vi "HTSuperProWriteControl.vi"(0 "Digital Control":u8, 3 "NXT":T1={"error"={"status"=FALSE, "code"=0, "source"=""}, "address"="", "NXT #"=-1, "Show Error"=TRUE, "Connection"=4} {"Connection" items=["USB", "Bluetooth", "USB then Bluetooth", "Last Connection", "Preference"]}, 4 "Port":T2 items=["Port 1", "Port 2", "Port 3", "Port 4"]) -> (5 "NXT":T1={"error"={"status"=FALSE, "code"=0, "source"=""}, "address"="", "NXT #"=-1, "Show Error"=TRUE, "Connection"=4} {"Connection" items=["USB", "Bluetooth", "USB then Bluetooth", "Last Connection", "Preference"]})   [LabVIEW 2009]
doc: "HiTechnic SuperPro - Write Control\n\n<B>Inputs\nPort </B> is the port connected to the sensor. Port 1 is the default, but Port 2, Port 3, or Port 4 can also be selected.\n<B>NXT </B> connects to NXT terminal of previous VI to establish the flow of the program.\n<B>Digital Control</B> bits set to 1 in the Digital Control will configure corresponding output B0-B7 pins as output. By default all pins on the SuperPro are set for input.\n\n<B>Outputs\nNXT </B> wires to NXT terminal of next VI to establish the flow of the program."
uses:
  <vilib>/NXT/Block Support/NXT_InputPort.ctl
  <vilib>/NXT/Subs/LVHSConnector.ctl
  <vilib>/NXT/Block Support/HWPage.SensorType.ctl
  <vilib>/NXT/Block Support/HWPage.SensorMode.ctl
panel:
  # "HiTechnic SuperPro Prototype board VI\nWrite Control\n\nBits set to 1 in the Digital Control will configure corresponding output B0-B7 pins as output.   By default all pins on the SuperPro are set for input.\n\n(c) HiTechnic 2011"
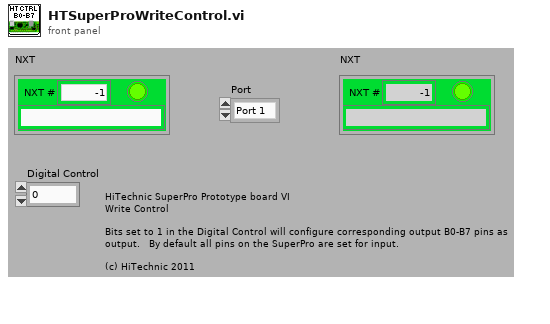
[diagram p1: front panel]
types:
  T1 = typedef "LVHSConnector.ctl" = cluster{"error":errorcluster, "address":string, "NXT #":i32, "Show Error":bool, "Connection":u16}
  T2 = typedef "NXT_InputPort.ctl" = u8
  T3 = typedef "HWPage.SensorType.ctl" = u8
  T4 = typedef "HWPage.SensorMode.ctl" = u8
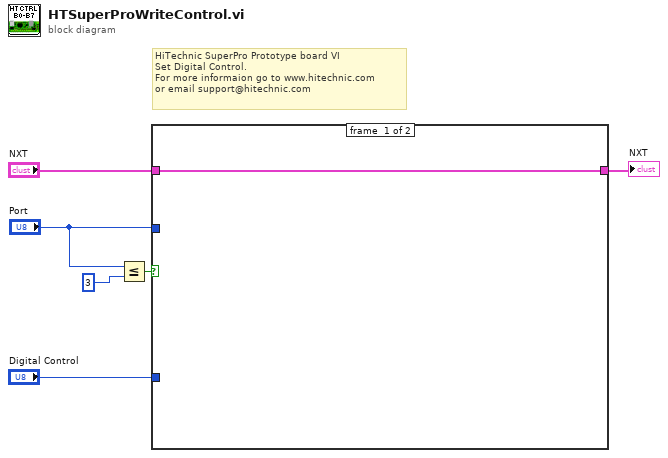
[diagram p0: block diagram]
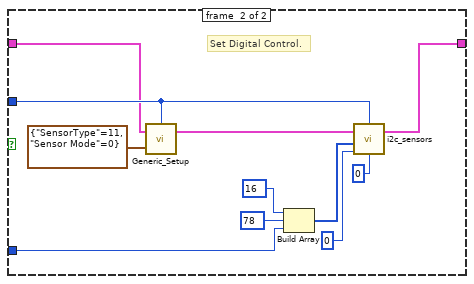
[diagram p2: hidden frame]
diagram:
  # "HiTechnic SuperPro Prototype board VI\nSet Digital Control.\nFor more informaion go to www.hitechnic.com\nor email support@hitechnic.com"
  n1 = Less Or Equal?(x="Port", y=u8 3) -> (x <= y?=w2:bool)
  n2 = case shown="True" w2 {
    tunnel: "Port" -> [_ w17]
    tunnel: "NXT" -> [w7 w16]
    tunnel: [w7 w14] -> w4
    tunnel: "Digital Control" -> [_ w9]
    frame #0 {
    }
    frame #1 {
      # "Set Digital Control."
      n3 = call <vilib>:"Generic_Setup.vi"("Sensor Setup"=cluster{"SensorType":T3, "Sensor Mode":T4} {"SensorType"=11, "Sensor Mode"=0}, "NXT"=w16, "Port"=w17) -> ("NXT"=w15:T1)  [unwired: 1 out]
      n4 = Build Array(u8 16, u8 78, w9) -> (w12:u8[])
      n5 = call <vilib>:"i2c_sensors.vi"("Return Length"=u8 0, "Bytes to Write"=w12, "Wait (msec)"=u32 0, "NXT"=w15, "Port"=w17) -> ("NXT"=w14:T1)  [unwired: 2 out]
    }
  }
  "NXT" <- w4
